vi "H5Pset_external.vi"(5 "Offset":i32, 6 "error in (no error)":errorcluster, 7 "Size (Unlimited)":u64=18446744073709551615 format="%.0x", 8 "File":path, 9 "HDF5 Property Ref":T1) -> (0 "error out":errorcluster, 3 "HDF5 Ref out":T1)   [LabVIEW 2017]
doc: "Adds an external file to the list of external files."
uses:
  <vilib>/UPVI/lvhdf5/library.llb/HDF5 Ref.ctl
  <vilib>/UPVI/lvhdf5/hdf5.dll
panel:
  # "LVHDF5 Toolkit\nCopyright (c) 2005-2013 by Jason D. Sommerville\nCopyright (c) 2014 by UPVI, LLC.\n\nThis use and distribution of this file is governed by the terms found in \nLICENSE.txt distributed with this toolkit and installed at\n <user.lib>\\_lvhdf5\\LICENSE.txt"
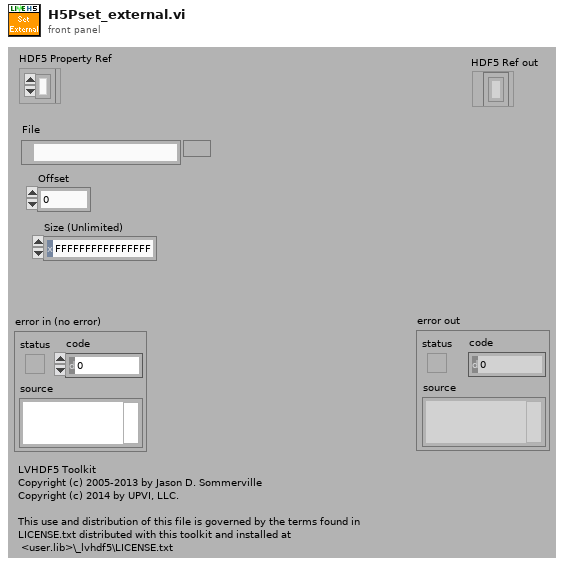
[diagram p1: front panel]
types:
  T1 = typedef "HDF5 Ref.ctl" = refnum<k1>
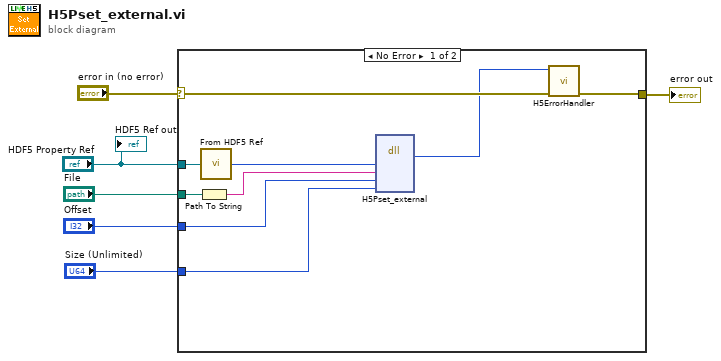
[diagram p0: block diagram]
diagram:
  n1 = case shown="No Error" "error in (no error)" {
    selector: "error in (no error)" -> [w15 w16]
    tunnel: [w14 w16] -> w5
    tunnel: "HDF5 Property Ref" -> [w12 _]
    tunnel: "File" -> [w10 _]
    tunnel: "Offset" -> [w8 _]
    tunnel: "Size (Unlimited)" -> [w7 _]
    frame No Error {
      n2 = Path To String(path=w10) -> (string=w9:string)
      n3 = call <vilib>:"From HDF5 Ref.vi"("HDF5 Ref"=w12) -> ("I32"=w11:i32)
      n4 = dll-call lib="C:/Program Files/National Instruments/LabVIEW 2017/vi.lib/UPVI/lvhdf5/hdf5.dll" fn="H5Pset_external"("plist_id"=w11, "name"=w9, "offset"=w8, "size"=w7) -> ("return type"=w13:i32)  [unwired: 7 in, 2 out]
      n5 = call <vilib>:"H5ErrorHandler.vi"("error in (no error)"=w15, "herr_t"=w13) -> ("error out"=w14:errorcluster)  [unwired: 3 in, 4 out]
    }
    frame Error {
    }
  }
  "error out" <- w5
  "HDF5 Ref out" <- "HDF5 Property Ref"
